vi "CANOpen_Format SDO to String Array.vi"(7 "Format":T1, 8 "error in (no error)":errorcluster, 11 "SDO Parameters":T2[](array[typedef]) {"Sub-Index (0)" format="%.0x"; "Object Index" format="%.0x"; "Block Data" format="%.0x"}) -> (0 "error out":errorcluster, 3 "Array":string[][](array[string]))   [LabVIEW 2013]
uses:
  Shared Code/CANOpen_SDO Settings.ctl
  CANOpen_SDO data format.ctl
  CANOpen Addon Custom Device.lvlib
panel:
  # "LSB"
  # "MSB"
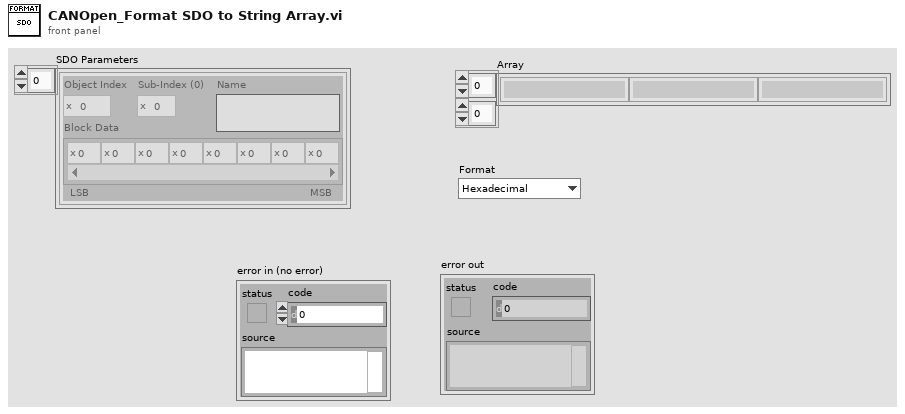
[diagram p1: front panel]
types:
  T1 = typedef "CANOpen Addon Custom Device.lvlib/CANOpen_SDO data format.ctl" = enum16{"Hexadecimal", "Decimal"}
  T2 = typedef "CANOpen Addon Custom Device.lvlib/CANOpen_SDO Settings.ctl" = cluster{"Object Index":u16, "Sub-Index (0)":u8, "Block Data":u8[], "Name":string}
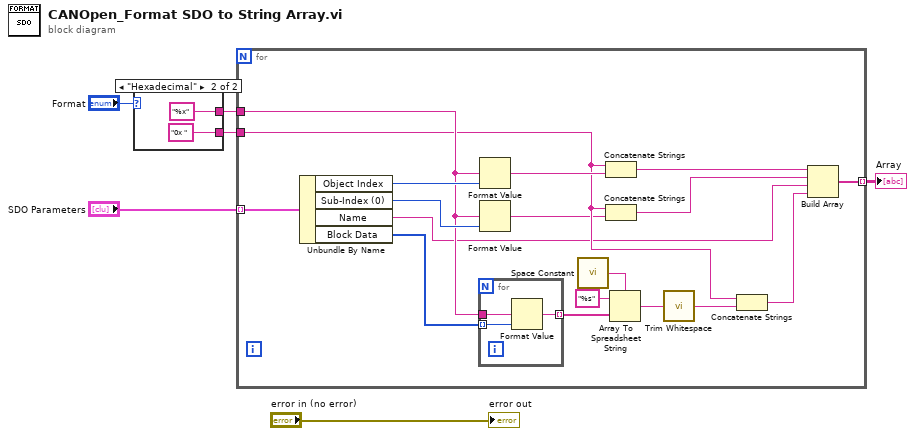
[diagram p0: block diagram]
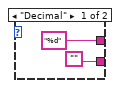
[diagram p2: hidden frame]
diagram:
  n1 = case shown="\"Hexadecimal\"" "Format" {
    tunnel: ["%d" "%x"] -> w5
    tunnel: ["" "0x "] -> w1
    frame "Decimal" {
    }
    frame "Hexadecimal" {
    }
  }
  n2 = for {
    tunnel: "SDO Parameters" -> [w28] mode=indexing
    tunnel: w5 -> [w18]
    tunnel: [w21] -> w3 mode=indexing
    tunnel: w1 -> [w15]
    n3 = Unbundle By Name(w28) -> ("Object Index"=w26:u16, "Sub-Index (0)"=w27:u8, "Name"=w12:string, "Block Data"=w13:u8[])
    n4 = for {
      tunnel: w13 -> [w31] mode=indexing
      tunnel: w18 -> [w30]
      tunnel: [w29] -> w25 mode=indexing
      n5 = Format Value(format string=w30, value (0)=w31) -> (output string=w29:string)  [unwired: 1 in]
    }
    n6 = Format Value(format string=w18, value (0)=w26) -> (output string=w19:string)  [unwired: 1 in]
    n7 = Format Value(format string=w18, value (0)=w27) -> (output string=w14:string)  [unwired: 1 in]
    n8 = call <vilib>:"Space Constant.vi"() -> ("String"=w23:string)
    n9 = Concatenate Strings(w15, w19) -> (w20:string)
    n10 = Concatenate Strings(w15, w14) -> (w17:string)
    n11 = Array To Spreadsheet String(delimiter (Tab)=w23, array=w25, 3:"%s" ("format string")) -> (spreadsheet string=w22:string)
    n12 = call <vilib>:"Trim Whitespace.vi"("string"=w22) -> ("trimmed string"=w16:string)  [unwired: 1 in]
    n13 = Concatenate Strings(w15, w16) -> (w11:string)
    n14 = Build Array(w20, w17, w12, w11) -> (w21:string[])
  }
  "Array" <- w3
  "error out" <- "error in (no error)"
